vi "read keyword.vi"(8 "error in (no error)":errorcluster, 10 "keyword":string, 11 "Simulated_Header in":refnum<class "Simulated_Header.lvclass">) -> (0 "error out":errorcluster, 2 "value":string, 3 "Simulated_Header out":refnum<class "Simulated_Header.lvclass">)   [LabVIEW 2018, in "Simulated_Header.lvclass"]
uses:
  Simulated_Header.lvclass
  Simulated_Header.lvclass/Simulated_Header.ctl
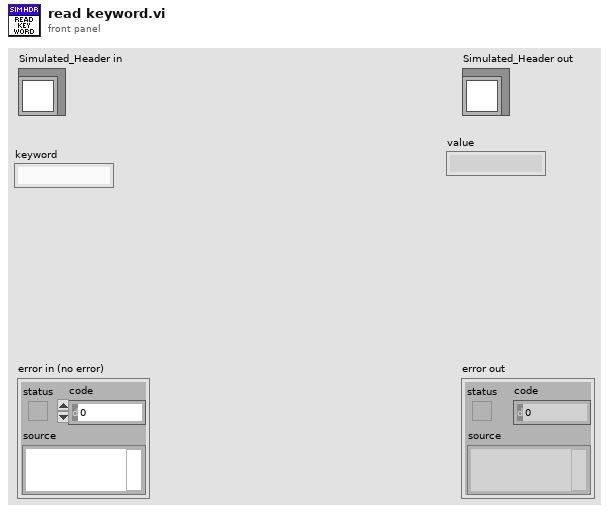
[diagram p1: front panel]
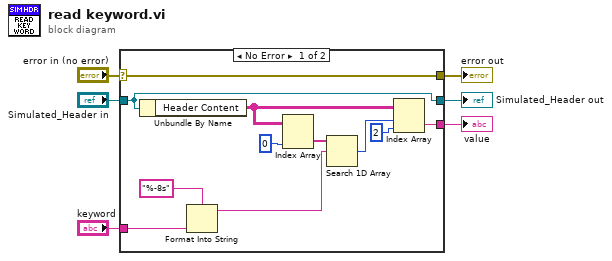
[diagram p0: block diagram]
diagram:
  n1 = case shown="No Error" "error in (no error)" {
    selector: "error in (no error)" -> [w17 w19]
    tunnel: [w17 w19] -> w5
    tunnel: [w16 w18] -> w3
    tunnel: "Simulated_Header in" -> [w16 w18]
    tunnel: "keyword" -> [w8 _]
    tunnel: [w10 _] -> w1
    frame No Error {
      n2 = Unbundle By Name(w16) -> ("Header Content"=w13:string[][])
      n3 = Format Into String(format string="%-8s", w8) -> (resulting string=w7:string)  [unwired: 2 in, 1 out]
      n4 = Index Array(array=w13, index (col)=0 ("disabled index (col)")) -> (element=w15:string[])  [unwired: 1 in]
      n5 = Search 1D Array(1D array=w15, element=w7) -> (index of element=w12:i32)  [unwired: 1 in]
      n6 = Index Array(array=w13, index (row)=w12, index (col)=2 ("disabled index (col)")) -> (element=w10:string)
    }
    frame Error {
    }
  }
  "error out" <- w5
  "Simulated_Header out" <- w3
  "value" <- w1
